vi "Abstract Message Name Dialog.vi"(8 "Start Path":path) -> (0 "Path out":path, 1 "Cancelled?":bool, 2 "Name":string, 3 "Use Reference Method out":bool)   [LabVIEW 2020, in "Actor Message Maker Provider.lvlib"]
uses:
  Actor Message Maker Provider.lvlib
  MessageMakerProvider/Support/Localized Strings.vi
  MessageMakerProvider/Message Maker Provider.lvlib
panel:
  out "Path Display":string
  in  "Path":path caption="Select a path to the reference method."
  in  "Use Reference Method":bool
  in  "Cancel Button":bool
  in  "OK Button":bool
  in  "Name":string caption="Enter a name for the new message."
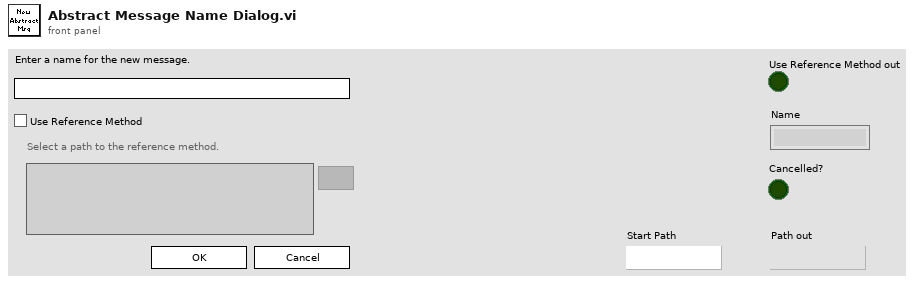
[diagram p1: front panel]
types:
  T1 = enum8{"Enabled", "Disabled", "Disabled and Grayed Out"}
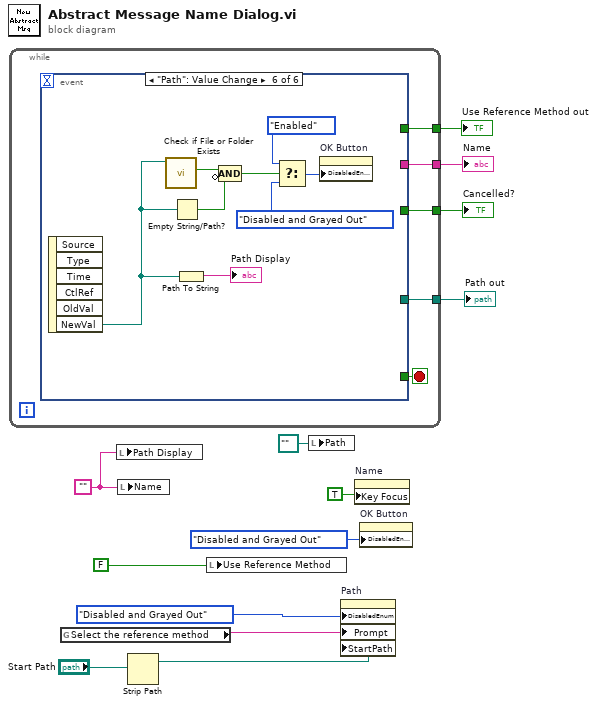
[diagram p0: block diagram]
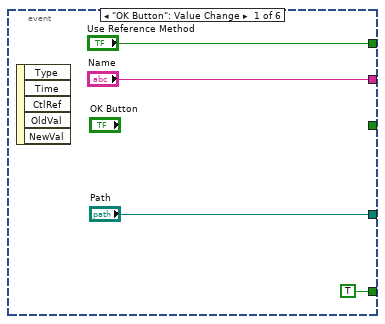
[diagram p2: hidden frame]
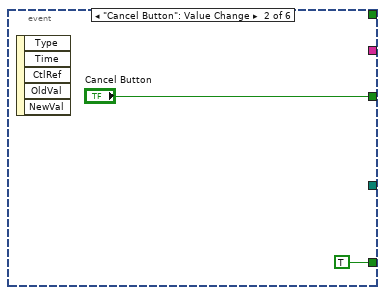
[diagram p3: hidden frame]
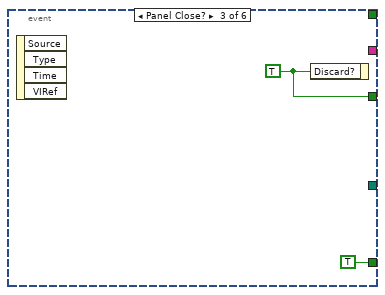
[diagram p4: hidden frame]
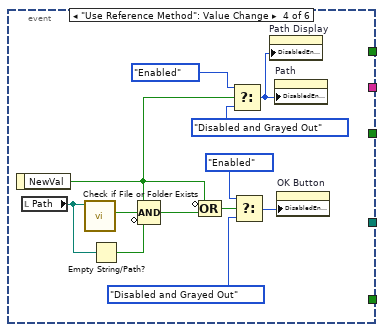
[diagram p5: hidden frame]
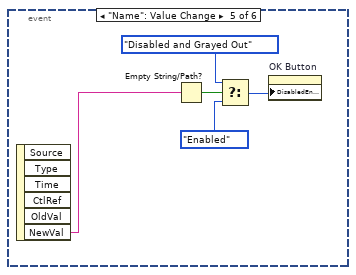
[diagram p6: hidden frame]
diagram:
  w3 = "" ("Name")
  n1 = while {
    tunnel: [w18] -> w13
    tunnel: [w17] -> w12
    tunnel: [w16] -> w10
    tunnel: [w15] -> w8
    stop <- w14 stop-if-true
    n2 = event shown="[5] \"Path\": Value Change" {
      selector: _ -> [_ _ _ _ _ _]
      dyn-events: _ -> [_ _ _ _ _ _]
      timeout: _ -> [_ _ _ _ _ _]
      tunnel: ["Name" _ _ _ _ _] -> w18
      tunnel: [_ "Cancel Button" w26 _ _ _] -> w17
      tunnel: ["Use Reference Method" _ _ _ _ _] -> w16
      tunnel: ["Path" _ _ _ _ _] -> w15
      tunnel: [TRUE TRUE TRUE _ _ _] -> w14
      event "OK Button": Value Change {
        n3 = event-data() -> ()  [unwired: 1 in, 5 out]
      }
      event "Cancel Button": Value Change {
        n4 = event-data() -> ()  [unwired: 1 in, 5 out]
      }
      event Panel Close? {
        w26 = TRUE ("Discard?")
        n5 = event-data() -> ()  [unwired: 1 in, 4 out]
        n6 = event-data("Discard?"=w26) -> ()  [unwired: 1 in, 1 out]
      }
      event "Use Reference Method": Value Change {
        n7 = event-data() -> ("NewVal"=w28:bool)  [unwired: 1 in]
        n8 = local read "Path"() -> (w30:path)
        n9 = call <vilib>:"Check if File or Folder Exists.vi"("path"=w30) -> ("file or folder exists?"=w31:bool)  [unwired: 8 in, 2 out]
        n10 = Empty String/Path?(string/path=w30) -> (empty?=w29:bool)
        n11 = Compound Arithmetic op=AND(w28, w31, invert w29) -> (w33:bool)
        n12 = Compound Arithmetic op=OR(invert w28, w33) -> (w32:bool)
        n13 = Select(t=T1."Enabled", s=w28, f=T1."Disabled and Grayed Out" ("Disabled")) -> (s? t:f=w27:T1)
        n14 = Select(t=T1."Enabled", s=w32, f=T1."Disabled and Grayed Out" ("Disabled")) -> (s? t:f=w36:T1)
        n15 = property on="Path Display" class="Str"("DisabledEnum"=w27) -> ()  [unwired: 2 in, 2 out]
        n16 = property on="Path" class="Path"("DisabledEnum"=w27) -> ()  [unwired: 2 in, 2 out]
        n17 = property on="OK Button" class="Bool"("DisabledEnum"=w36) -> ()  [unwired: 2 in, 2 out]
      }
      event "Name": Value Change {
        n18 = event-data() -> ("NewVal"=w39:string)  [unwired: 1 in, 5 out]
        n19 = Empty String/Path?(string/path=w39) -> (empty?=w40:bool)
        n20 = Select(t=T1."Disabled and Grayed Out", s=w40, f=T1."Enabled" ("Disabled")) -> (s? t:f=w41:T1)
        n21 = property on="OK Button" class="Bool"("DisabledEnum"=w41) -> ()  [unwired: 2 in, 2 out]
      }
      event "Path": Value Change {
        n22 = event-data() -> ("NewVal"=w44:path)  [unwired: 1 in, 5 out]
        n23 = call <vilib>:"Check if File or Folder Exists.vi"("path"=w44) -> ("file or folder exists?"=w48:bool)  [unwired: 8 in, 2 out]
        n24 = Empty String/Path?(string/path=w44) -> (empty?=w47:bool)
        n25 = Path To String(path=w44) -> (string=→"Path Display":string)
        n26 = Compound Arithmetic op=AND(w48, invert w47) -> (w46:bool)
        n27 = Select(t=T1."Enabled", s=w46, f=T1."Disabled and Grayed Out" ("Disabled")) -> (s? t:f=w51:T1)
        n28 = property on="OK Button" class="Bool"("DisabledEnum"=w51) -> ()  [unwired: 2 in, 2 out]
      }
    }
  }
  "Name" <- w13
  "Cancelled?" <- w12
  "Use Reference Method out" <- w10
  "Path out" <- w8
  n29 = global read "Localized Strings.vi" "Select the reference method"() -> (w6:string)
  n30 = local write "Path Display"(w3) -> ()
  n31 = local write "Name"(w3) -> ()
  n32 = Strip Path(path="Start Path") -> (stripped path=w4:path)  [unwired: 1 out]
  n33 = local write "Use Reference Method"(FALSE ("Use Reference Method")) -> ()
  n34 = local write "Path"(path "" ("Path")) -> ()
  n35 = property on="Path" class="Path"("DisabledEnum"=T1."Disabled and Grayed Out" ("Disabled"), "Prompt"=w6, "StartPath"=w4) -> ()  [unwired: 2 in, 2 out]
  n36 = property on="Name" class="Str"("Key Focus"=TRUE) -> ()  [unwired: 2 in, 2 out]
  n37 = property on="OK Button" class="Bool"("DisabledEnum"=T1."Disabled and Grayed Out" ("Disabled")) -> ()  [unwired: 2 in, 2 out]
